vi "ep_Complex Spectra Calculation.vi"(0 "data in":dbl[](array[numeric]), 1 "df":dbl, 2 "f0":dbl, 5 "algorithm":enum16{"Average", "RMS"}(ring), 7 "aggregated data valid? (F)":bool, 9 "restart aggregation? (F)":bool, 11 "error in (no error)":errorcluster, 12 "aggregated data":T1, 13 "runs":u32) -> (4 "aggregated minimum values":cluster{"f0":dbl, "df":dbl, "amplitudes":dbl[]}, 6 "aggregated avgeraged/RMS values":cluster{"f0":dbl, "df":dbl, "amplitudes":dbl[]}, 8 "aggregated maximum values":cluster{"f0":dbl, "df":dbl, "amplitudes":dbl[]}, 14 "aggregated data":T1, 15 "error out":errorcluster)   [LabVIEW 2014, in "NI_EP_Power Quality.lvlib"]
doc: "Calculates the aggregated minimum, maximum, and averaged or RMS value of an input signal for a specified aggregation interval, according to Class S in IEC 61000-4-30:2008. There is no overlap between aggregation intervals. This VI automatically restarts accumulation at the beginning of the next time interval after the previous interval expires. You must manually select the polymorphic instance you want to use."
uses:
  <vilib>/addons/Electrical Power/PQ/NI_EP_Power Quality.lvlib
  <vilib>/addons/Electrical Power/PQ/Common/Controls/ep_Aggregation Data.ctl
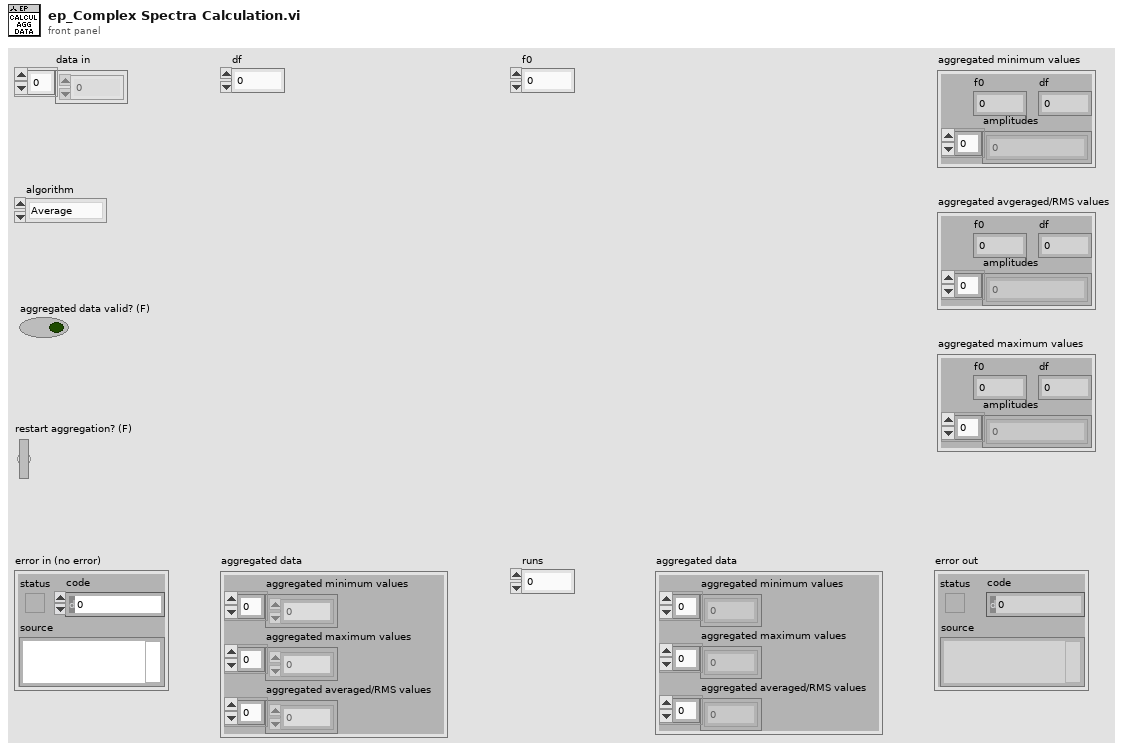
[diagram p1: front panel]
types:
  T1 = typedef "NI_EP_Power Quality.lvlib/ep_Aggregation Data.ctl" = cluster{"aggregated minimum values":dbl[], "aggregated maximum values":dbl[], "aggregated averaged/RMS values":dbl[]}
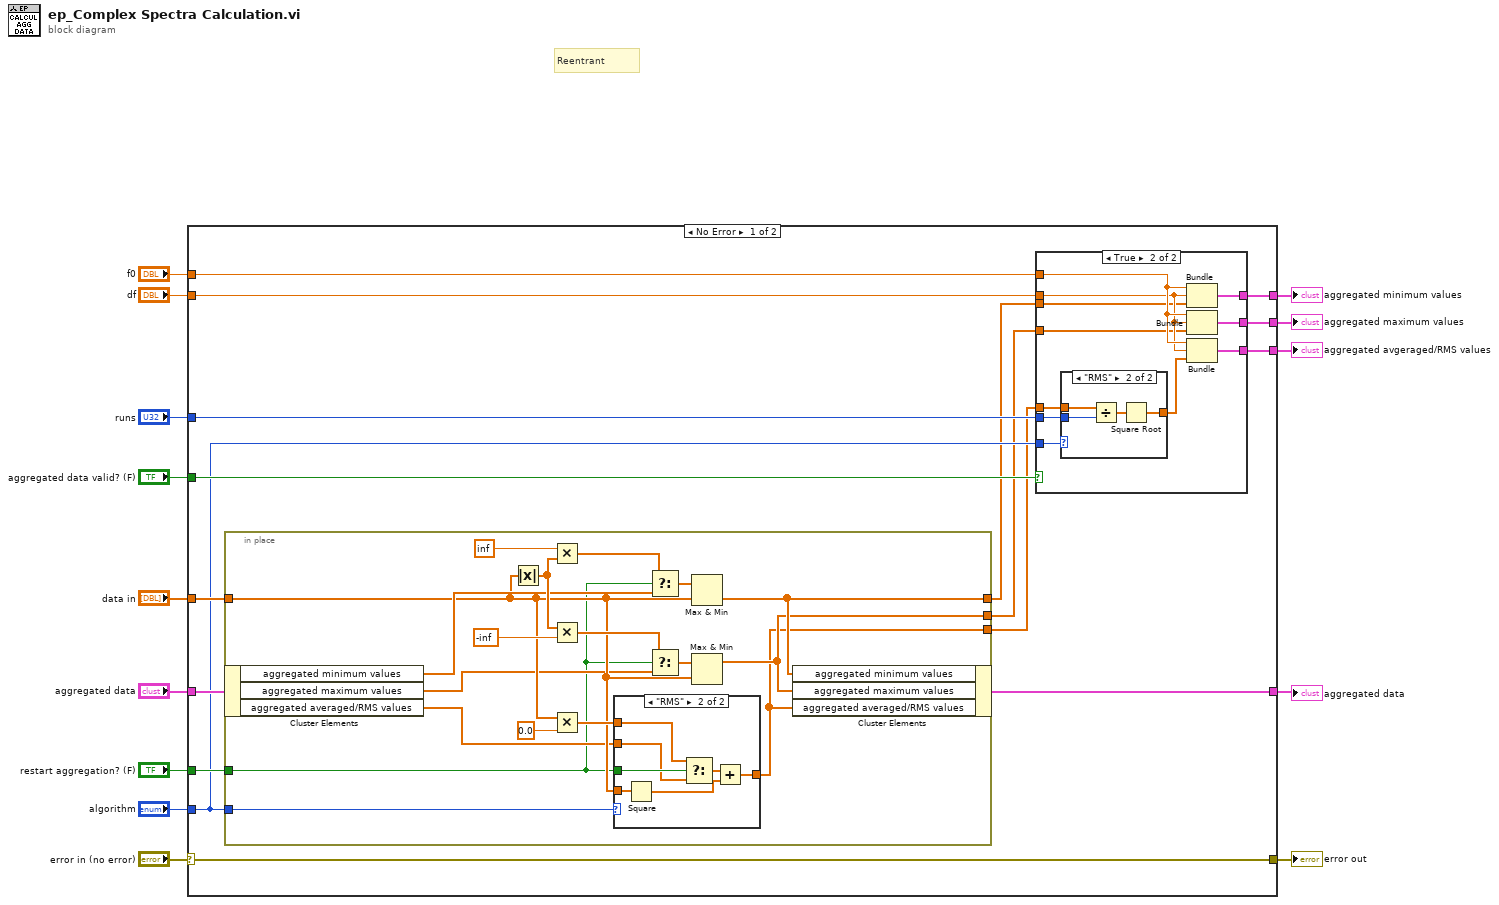
[diagram p0: block diagram]
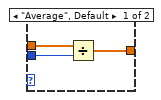
[diagram p3: hidden frame]
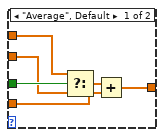
[diagram p4: hidden frame]
diagram:
  # "Reentrant"
  n1 = case shown="No Error" "error in (no error)" {
    selector: "error in (no error)" -> [w18 w80]
    tunnel: "aggregated data" -> [w30 _]
    tunnel: "data in" -> [w29 _]
    tunnel: "restart aggregation? (F)" -> [w28 _]
    tunnel: "aggregated data valid? (F)" -> [w27 _]
    tunnel: "f0" -> [w26 _]
    tunnel: "df" -> [w25 _]
    tunnel: [w24 _] -> w8
    tunnel: [w23 _] -> w7
    tunnel: "runs" -> [w22 _]
    tunnel: [w21 _] -> w5
    tunnel: [w20 _] -> w4
    tunnel: "algorithm" -> [w19 _]
    tunnel: [w18 w80] -> w1
    frame No Error {
      n2 = in-place {
        in-place-border: w29 -> [w56]
        in-place-border: w28 -> [w53]
        in-place-border: w19 -> [w52]
        in-place-border: [w51] -> w17
        in-place-border: [w50] -> w16
        in-place-border: [w49] -> w15
        n3 = in-place-cluster #1(w30) -> ("aggregated minimum values"=w57:dbl[], "aggregated maximum values"=w55:dbl[], "aggregated averaged/RMS values"=w54:dbl[])
        n4 = Absolute Value(x=w56) -> (abs(x)=w66:dbl[])
        n5 = Multiply(x=inf, y=w66) -> (x*y=w61:dbl[])
        n6 = Multiply(x=w66, y=-inf) -> (x*y=w63:dbl[])
        n7 = Multiply(x=w56, y=0.0) -> (x*y=w65:dbl[])
        n8 = case shown="\"RMS\"" w52 {
          tunnel: w56 -> [w70 w77]
          tunnel: w53 -> [w71 w78]
          tunnel: w65 -> [w69 w75]
          tunnel: w54 -> [w68 w74]
          tunnel: [w67 w73] -> w49
          frame "Average", Default {
            n9 = Select(t=w69, s=w71, f=w68) -> (s? t:f=w72:dbl[])
            n10 = Add(x=w72, y=w70) -> (x+y=w67:dbl[])
          }
          frame "RMS" {
            n11 = Square(x=w77) -> (x^2=w76:dbl[])
            n12 = Select(t=w75, s=w78, f=w74) -> (s? t:f=w79:dbl[])
            n13 = Add(x=w79, y=w76) -> (x+y=w73:dbl[])
          }
        }
        n14 = Select(t=w61, s=w53, f=w57) -> (s? t:f=w58:dbl[])
        n15 = Select(t=w63, s=w53, f=w55) -> (s? t:f=w59:dbl[])
        n16 = Max & Min(x=w58, y=w56) -> (min(x,y)=w51:dbl[])  [unwired: 1 out]
        n17 = Max & Min(x=w59, y=w56) -> (max(x,y)=w50:dbl[])  [unwired: 1 out]
        n18 = in-place-cluster #1("aggregated minimum values"=w51, "aggregated maximum values"=w50, "aggregated averaged/RMS values"=w49) -> (w20:T1)
      }
      n19 = case shown="True" w27 {
        tunnel: w26 -> [_ w41]
        tunnel: w25 -> [_ w40]
        tunnel: [_ w39] -> w24
        tunnel: [_ w38] -> w23
        tunnel: [_ w37] -> w21
        tunnel: w19 -> [_ w36]
        tunnel: w22 -> [_ w35]
        tunnel: w17 -> [_ w33]
        tunnel: w16 -> [_ w32]
        tunnel: w15 -> [_ w31]
        frame False {
        }
        frame True {
          n20 = case shown="\"RMS\"" w36 {
            tunnel: w31 -> [w44 w48]
            tunnel: w35 -> [w43 w47]
            tunnel: [w42 w45] -> w34
            frame "Average", Default {
              n21 = Divide(x=w44, y=w43) -> (x/y=w42:dbl[])
            }
            frame "RMS" {
              n22 = Divide(x=w48, y=w47) -> (x/y=w46:dbl[])
              n23 = Square Root(x=w46) -> (sqrt(x)=w45:dbl[])
            }
          }
          n24 = Bundle("f0"=w41, "df"=w40, w33) -> (w39:cluster{"f0":dbl, "df":dbl, dbl[]})  [unwired: 1 in]
          n25 = Bundle("f0"=w41, "df"=w40, w32) -> (w38:cluster{"f0":dbl, "df":dbl, dbl[]})  [unwired: 1 in]
          n26 = Bundle("f0"=w41, "df"=w40, w34) -> (w37:cluster{"f0":dbl, "df":dbl, dbl[]})  [unwired: 1 in]
        }
      }
    }
    frame Error {
    }
  }
  "aggregated data" <- w4
  "aggregated minimum values" <- w8
  "aggregated avgeraged/RMS values" <- w5
  "aggregated maximum values" <- w7
  "error out" <- w1
